vi "Set Channel group.vi"(8 "error in (no error)":errorcluster, 10 "Channel group in":refnum<class "Channel group.lvclass">, 11 "FPGA Device in":refnum<class "FPGA Device.lvclass">) -> (0 "error out":errorcluster, 2 "replaced":bool, 3 "FPGA Device out":refnum<class "FPGA Device.lvclass">)   [LabVIEW 2016, in "FPGA RM Shared API.lvlib" / "FPGA Device.lvclass"]
uses:
  FPGA Device.lvclass
  Channel Group/Channel group.lvclass
  Channel Group/Channel group.lvclass/Channel group.ctl
  FPGA Device.lvclass/FPGA Device.ctl
  Channel Group/Read channel type.vi
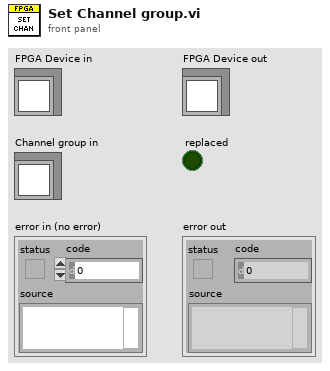
[diagram p1: front panel]
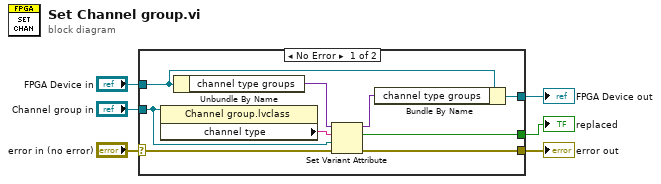
[diagram p0: block diagram]
diagram:
  n1 = case shown="No Error" "error in (no error)" {
    selector: "error in (no error)" -> [w11 w17]
    tunnel: [w10 w17] -> w5
    tunnel: [w14 w16] -> w3
    tunnel: "FPGA Device in" -> [w15 w16]
    tunnel: "Channel group in" -> [w8 _]
    tunnel: [w9 _] -> w1
    frame No Error {
      n2 = property class="Channel group.lvclass"(reference=w8) -> ("channel type"=w7:string)  [unwired: 1 in, 2 out]
      n3 = Unbundle By Name(w15) -> ("channel type groups"=w13:variant)
      n4 = Set Variant Attribute(Variant=w13, name=w7, value=w8, error in=w11) -> (Variant out=w12:variant, replaced=w9:bool, error out=w10:errorcluster)
      n5 = Bundle By Name(cluster=w15, "channel type groups"=w12) -> (w14:refnum<class "FPGA Device.lvclass">)
    }
    frame Error {
    }
  }
  "error out" <- w5
  "FPGA Device out" <- w3
  "replaced" <- w1
